vi "LINAKParseStopReason.vi"(11 "Numeric Control":u16) -> (3 "ReasonForLastStop":string)   [LabVIEW 2017]
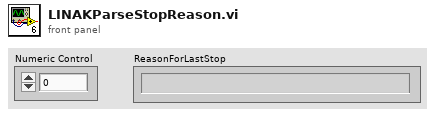
[diagram p1: front panel]
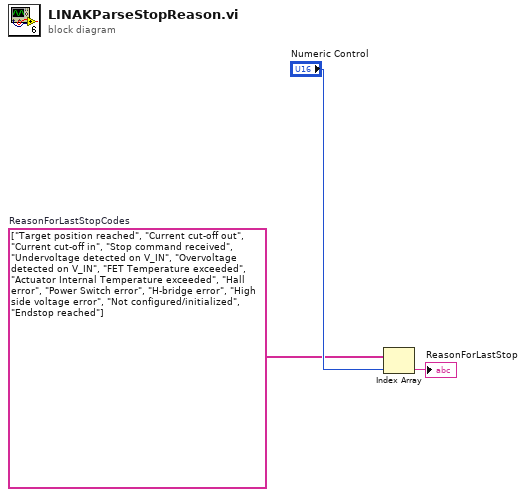
[diagram p0: block diagram]
diagram:
  w1 = string[] ["Target position reached", "Current cut-off out", "Current cut-off in", "Stop command received", "Undervoltage detected on V_IN", "Overvoltage detected on V_IN", "FET Temperature exceeded", "Actuator Internal Temperature exceeded", "Hall error", "Power Switch error", "H-bridge error", "High side voltage error", "Not configured/initialized", "Endstop reached"]  # ReasonForLastStopCodes
  n1 = Index Array(array=w1, index="Numeric Control") -> (element=→"ReasonForLastStop":string)
